vi "First_input_values.vi"() -> ()   [LabVIEW 2014]
panel:
  in  "Active":bool
  in  "Multi Values":dbl[][][](array[numeric])=[[[0.0, 0.0, 0.0, 0.0, 0.0, 0.0, 0.0], [0.01, 0.5, 0.5, 0.1, 0.01, 0.0, 0.0], [19.0, 15.0, 15.0, 25.0, 18.0, 0.0, 0.0], [0.0, 0.0, 0.0, 0.0, 0.0, 0.0, 0.0], [0.01, 0.5, 0.5, 0.1, 0.01, 0.0, 0.0], [19.0, 15.0, 15.0, 25.0, 18.0, 0.0, 0.0]], [[0.0, 0.0, 0.0, 0.0, 0.0, 0.0, 0.0], [0.01, 0.5, 0.5, 0.1, 0.01, 0.0, 0.0], [19.0, 19.0, 19.0, 25.0, 18.0, 0.0, 0.0], [0.0, 0.0, 0.0, 0.0, 0.0, 0.0, 0.0], [0.01, 0.5, 0.5, 0.1, 0.01, 0.0, 0.0], [19.0, 19.0, 19.0, 25.0, 18.0, 0.0, 0.0]], [[0.0, 0.0, 0.0, 0.0, 0.0, 0.0, 0.0], [0.01, 0.5, 0.5, 0.1, 0.01, 0.0, 0.0], [19.0, 19.0, 19.0, 25.0, 18.0, 0.0, 0.0], [0.0, 0.0, 0.0, 0.0, 0.0, 0.0, 0.0], [0.01, 0.5, 0.5, 0.1, 0.01, 0.0, 0.0], [19.0, 19.0, 19.0, 25.0, 18.0, 0.0, 0.0]], [[0.0, 0.0, 0.0, 0.0, 0.0, 0.0, 0.0], [0.01, 0.5, 0.5, 0.1, 0.01, 0.0, 0.0], [19.0, 19.0, 19.0, 25.0, 18.0, 0.0, 0.0], [0.0, 0.0, 0.0, 0.0, 0.0, 0.0, 0.0], [0.01, 0.5, 0.5, 0.1, 0.01, 0.0, 0.0], [19.0, 19.0, 19.0, 25.0, 18.0, 0.0, 0.0]], [[0.0, 0.0, 0.0, 0.0, 0.0, 0.0, 0.0], [0.01, 0.5, 0.5, 0.1, 0.01, 0.0, 0.0], [19.0, 19.0, 19.0, 25.0, 18.0, 0.0, 0.0], [0.0, 0.0, 0.0, 0.0, 0.0, 0.0, 0.0], [0.01, 0.5, 0.5, 0.1, 0.01, 0.0, 0.0], [19.0, 19.0, 19.0, 25.0, 18.0, 0.0, 0.0]], [[0.0, 0.0, 0.0, 0.0, 0.0, 0.0, 0.0], [0.01, 0.5, 0.5, 0.1, 0.01, 0.0, 0.0], [19.0, 19.0, 19.0, 25.0, 18.0, 0.0, 0.0], [0.0, 0.0, 0.0, 0.0, 0.0, 0.0, 0.0], [0.01, 0.5, 0.5, 0.1, 0.01, 0.0, 0.0], [19.0, 19.0, 19.0, 25.0, 18.0, 0.0, 0.0]], [[0.0, 0.0, 0.0, 0.0, 0.0, 0.0, 0.0], [0.01, 0.5, 0.5, 0.1, 0.01, 0.0, 0.0], [19.0, 19.0, 19.0, 25.0, 18.0, 0.0, 0.0], [0.0, 0.0, 0.0, 0.0, 0.0, 0.0, 0.0], [0.01, 0.5, 0.5, 0.1, 0.01, 0.0, 0.0], [19.0, 19.0, 19.0, 25.0, 18.0, 0.0, 0.0]], [[0.0, 0.0, 0.0, 0.0, 0.0, 0.0, 0.0], [0.01, 0.5, 0.5, 0.1, 0.01, 0.0, 0.0], [19.0, 16.0, 16.0, 25.0, 18.0, 0.0, 0.0], [0.0, 0.0, 0.0, 0.0, 0.0, 0.0, 0.0], [0.01, 0.5, 0.5, 0.1, 0.01, 0.0, 0.0], [19.0, 16.0, 16.0, 25.0, 18.0, 0.0, 0.0]], [[0.0, 0.0, 0.0, 0.0, 0.0, 0.0, 0.0], [0.0, 0.0, 0.0, 0.0, 0.0, 0.0, 0.0], [0.0, 0.0, 0.0, 0.0, 0.0, 0.0, 0.0], [0.0, 0.0, 0.0, 0.0, 0.0, 0.0, 0.0], [0.0, 0.0, 0.0, 0.0, 0.0, 0.0, 0.0], [0.0, 0.0, 0.0, 0.0, 0.0, 0.0, 0.0]], [[0.0, 0.0, 0.0, 0.0, 0.0, 0.0, 0.0], [0.0, 0.0, 0.0, 0.0, 0.0, 0.0, 0.0], [0.0, 0.0, 0.0, 0.0, 0.0, 0.0, 0.0], [0.0, 0.0, 0.0, 0.0, 0.0, 0.0, 0.0], [0.0, 0.0, 0.0, 0.0, 0.0, 0.0, 0.0], [0.0, 0.0, 0.0, 0.0, 0.0, 0.0, 0.0]], [[0.0, 0.0, 0.0, 0.0, 0.0, 0.0, 0.0], [0.0, 0.0, 0.0, 0.0, 0.0, 0.0, 0.0], [0.0, 0.0, 0.0, 0.0, 0.0, 0.0, 0.0], [0.0, 0.0, 0.0, 0.0, 0.0, 0.0, 0.0], [0.0, 0.0, 0.0, 0.0, 0.0, 0.0, 0.0], [0.0, 0.0, 0.0, 0.0, 0.0, 0.0, 0.0]], [[0.0, 0.0, 0.0, 0.0, 0.0, 0.0, 0.0], [0.0, 0.0, 0.0, 0.0, 0.0, 0.0, 0.0], [0.0, 0.0, 0.0, 0.0, 0.0, 0.0, 0.0], [0.0, 0.0, 0.0, 0.0, 0.0, 0.0, 0.0], [0.0, 0.0, 0.0, 0.0, 0.0, 0.0, 0.0], [0.0, 0.0, 0.0, 0.0, 0.0, 0.0, 0.0]], [[0.0, 0.0, 0.0, 0.0, 0.0, 0.0, 0.0], [0.0, 0.0, 0.0, 0.0, 0.0, 0.0, 0.0], [0.0, 0.0, 0.0, 0.0, 0.0, 0.0, 0.0], [0.0, 0.0, 0.0, 0.0, 0.0, 0.0, 0.0], [0.0, 0.0, 0.0, 0.0, 0.0, 0.0, 0.0], [0.0, 0.0, 0.0, 0.0, 0.0, 0.0, 0.0]], [[0.0, 0.0, 0.0, 0.0, 0.0, 0.0, 0.0], [0.0, 0.0, 0.0, 0.0, 0.0, 0.0, 0.0], [0.0, 0.0, 0.0, 0.0, 0.0, 0.0, 0.0], [0.0, 0.0, 0.0, 0.0, 0.0, 0.0, 0.0], [0.0, 0.0, 0.0, 0.0, 0.0, 0.0, 0.0], [0.0, 0.0, 0.0, 0.0, 0.0, 0.0, 0.0]], [[0.0, 0.0, 0.0, 0.0, 0.0, 0.0, 0.0], [0.0, 0.0, 0.0, 0.0, 0.0, 0.0, 0.0], [0.0, 0.0, 0.0, 0.0, 0.0, 0.0, 0.0], [0.0, 0.0, 0.0, 0.0, 0.0, 0.0, 0.0], [0.0, 0.0, 0.0, 0.0, 0.0, 0.0, 0.0], [0.0, 0.0, 0.0, 0.0, 0.0, 0.0, 0.0]], [[0.0, 0.0, 0.0, 0.0, 0.0, 0.0, 0.0], [0.0, 0.0, 0.0, 0.0, 0.0, 0.0, 0.0], [0.0, 0.0, 0.0, 0.0, 0.0, 0.0, 0.0], [0.0, 0.0, 0.0, 0.0, 0.0, 0.0, 0.0], [0.0, 0.0, 0.0, 0.0, 0.0, 0.0, 0.0], [0.0, 0.0, 0.0, 0.0, 0.0, 0.0, 0.0]], [[0.0, 0.0, 0.0, 0.0, 0.0, 0.0, 0.0], [0.0, 0.0, 0.0, 0.0, 0.0, 0.0, 0.0], [0.0, 0.0, 0.0, 0.0, 0.0, 0.0, 0.0], [0.0, 0.0, 0.0, 0.0, 0.0, 0.0, 0.0], [0.0, 0.0, 0.0, 0.0, 0.0, 0.0, 0.0], [0.0, 0.0, 0.0, 0.0, 0.0, 0.0, 0.0]], [[0.0, 0.0, 0.0, 0.0, 0.0, 0.0, 0.0], [0.0, 0.0, 0.0, 0.0, 0.0, 0.0, 0.0], [0.0, 0.0, 0.0, 0.0, 0.0, 0.0, 0.0], [0.0, 0.0, 0.0, 0.0, 0.0, 0.0, 0.0], [0.0, 0.0, 0.0, 0.0, 0.0, 0.0, 0.0], [0.0, 0.0, 0.0, 0.0, 0.0, 0.0, 0.0]], [[0.0, 0.0, 0.0, 0.0, 0.0, 0.0, 0.0], [0.0, 0.0, 0.0, 0.0, 0.0, 0.0, 0.0], [0.0, 0.0, 0.0, 0.0, 0.0, 0.0, 0.0], [0.0, 0.0, 0.0, 0.0, 0.0, 0.0, 0.0], [0.0, 0.0, 0.0, 0.0, 0.0, 0.0, 0.0], [0.0, 0.0, 0.0, 0.0, 0.0, 0.0, 0.0]], [[0.0, 0.0, 0.0, 0.0, 0.0, 0.0, 0.0], [0.0, 0.0, 0.0, 0.0, 0.0, 0.0, 0.0], [0.0, 0.0, 0.0, 0.0, 0.0, 0.0, 0.0], [0.0, 0.0, 0.0, 0.0, 0.0, 0.0, 0.0], [0.0, 0.0, 0.0, 0.0, 0.0, 0.0, 0.0], [0.0, 0.0, 0.0, 0.0, 0.0, 0.0, 0.0]]]
  in  "Y range KV":dbl=19.0 min=0.0 max=26.0
  in  "Y range W":dbl=20.0 min=0.0 max=26.0
  in  "Y range 1R":dbl=21.0 min=0.0 max=26.0
  in  "Y range 10R":dbl=21.0 min=0.0 max=26.0
  in  "Y range AD":dbl=19.0 min=0.0 max=26.0
  in  "Y 2. input KV":dbl=0.01
  in  "Y 1. input KV":dbl
  in  "Y 2. input W":dbl=0.01
  in  "Y 1. input W":dbl
  in  "Y 2. input 1R":dbl=1.0
  in  "Y 1. input 1R":dbl
  in  "Y 2. input 10R":dbl=1.0
  in  "Y 1. input 10R":dbl
  in  "Y 2. input AD":dbl=0.01
  in  "Y 1. input AD":dbl
  in  "X range KV":dbl=19.0 min=0.0 max=26.0
  in  "X range W":dbl=25.0 min=0.0 max=26.0
  in  "X range 1R":dbl=21.0 min=0.0 max=26.0
  in  "X range 10R":dbl=21.0 min=0.0 max=26.0
  in  "X range AD":dbl=19.0 min=0.0 max=26.0
  in  "X 2. input KV":dbl=0.01
  in  "X 1. input KV":dbl
  in  "X 2. input W":dbl=0.1
  in  "X 1. input W":dbl
  in  "X 2. input 1R":dbl=1.0
  in  "X 1. input 1R":dbl
  in  "X 2. input 10R":dbl=1.0
  in  "X 1. input 10R":dbl
  in  "X 2. input AD":dbl=0.01
  in  "X 1. input AD":dbl
  # "Ok'un gösterdiği yeri arttırarak bir sonraki frekansın başlangıç değerlerini\ngirebilirsiniz."
  # "Eğer birden fazla frekans ile ölçüm alacaksanız sol tarafı aktif edin!"
  # "Array içine soldaki değerlerin sırasını bozmadan aynı şekilde girebilirsiniz."
  # "Tüm başlangıç değerlerini buradan giriniz"
  # "Input X 1 ->"
  # "Input X 2 ->"
  # "Range X (7-26) ->"
  # "Input XY 1 ->"
  # "Input XY 2 ->"
  # "Range Y (7-26) ->"
  # "Range (5) -> 100 nV"
  # "Range (13) -> 50 uV"
  # "Range (21) -> 20 mV"
  # "Range (6) -> 200 nV"
  # "Range (14) -> 100 uV"
  # "Range (22) -> 50 mV"
  # "Range (7) -> 500 nV"
  # "Range (15) -> 200 uV"
  # "Range (23) -> 100 mV"
  # "Range (8) -> 1 uV"
  # "Range (16) -> 500 uV"
  # "Range (24) -> 200 mV"
  # "Range (9) -> 2 uV"
  # "Range (17) -> 1 mV"
  # "Range (25) -> 500 mV"
  # "Range (10) -> 5 uV"
  # "Range (18) -> 2 mV"
  # "Range (26) -> 1 V"
  # "Range (11) -> 10 uV"
  # "Range (19) -> 5 mV"
  # "Range (26+) -> 1 V"
  # "Range (12) -> 20 uV"
  # "Range (20) -> 10 mV"
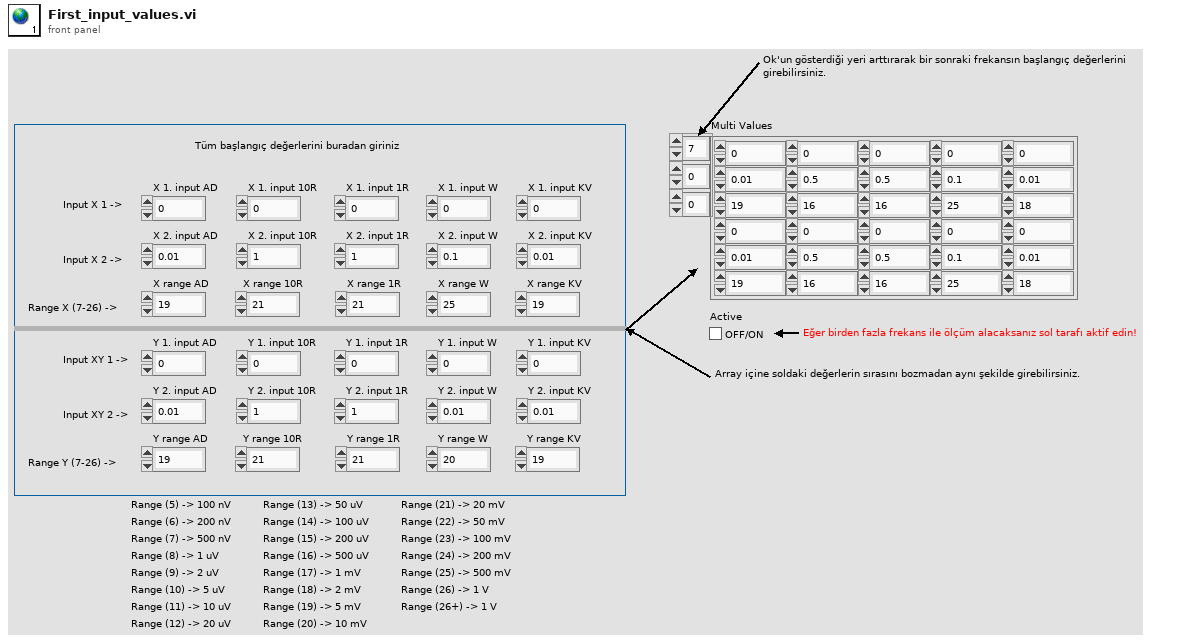
[diagram p1: front panel]
diagram:
